vi "Read Configuration File.vi"(8 "error in (no error)":errorcluster, 10 "Configuration filepath":string, 11 "TDCManager":T1) -> (0 "error out":errorcluster, 2 "Success?":bool, 3 "TDCManager":T1)   [LabVIEW 2016, in "HPTDC Driver Library.lvlib"]
uses:
  HPTDC Driver Library.lvlib
  Typedefs/TDCManager.ctl
  C:/Users/CRT Controller/CRTC Labview Application/Source/HPTDC Driver Library Folder/Library files/hptdc_net4_3.7.0_x64.dll
  hptdc_net4_3.7.0_x64.dll
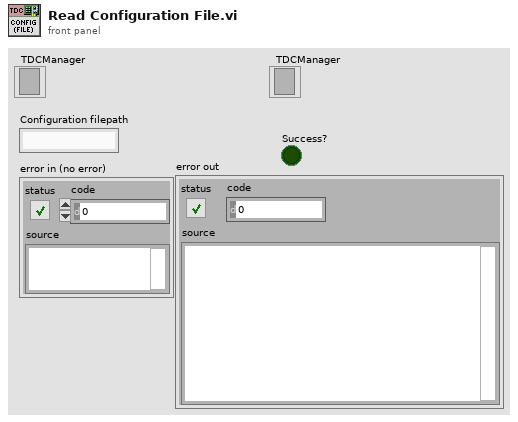
[diagram p1: front panel]
types:
  T1 = typedef "HPTDC Driver Library.lvlib/TDCManager.ctl" = refnum<k24>
  T2 = typedef "Semaphore RefNum" = refnum<k1>
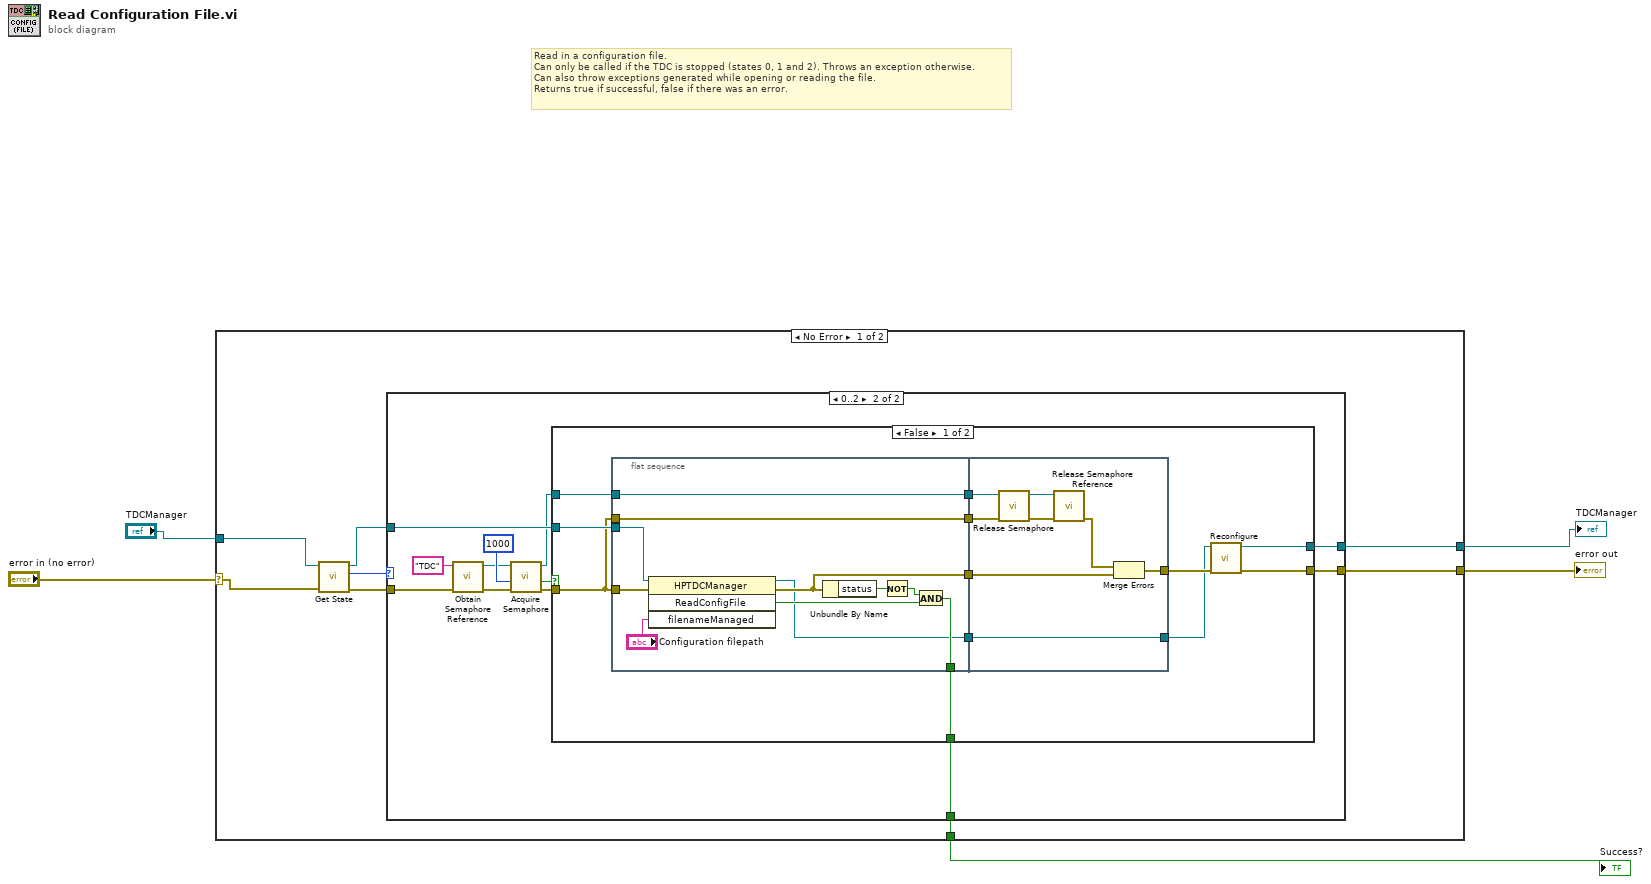
[diagram p0: block diagram]
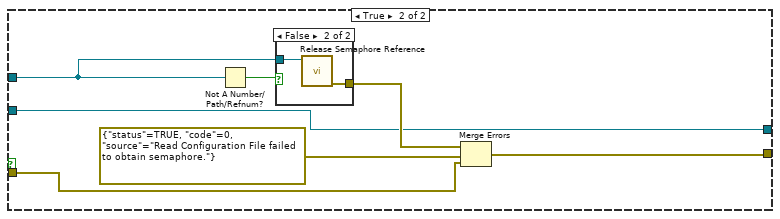
[diagram p3: hidden frame]
diagram:
  # "Read in a configuration file.\nCan only be called if the TDC is stopped (states 0, 1 and 2). Throws an exception otherwise.\nCan also throw exceptions generated while opening or reading the file.\nReturns true if successful, false if there was an error."
  n1 = case shown="No Error" "error in (no error)" {
    selector: "error in (no error)" -> [w6 w68]
    tunnel: [w10 w68] -> w5
    tunnel: [w9 _] -> w4
    tunnel: [w8 w69] -> w3
    tunnel: "TDCManager" -> [w7 w69]
    frame No Error {
      n2 = call "Get State.vi"("error in"=w6, "TDCManager"=w7) -> ("error out"=w11:errorcluster, "State"=w13:i32, "TDCManager"=w12:T1)  [unwired: 6 in, 1 out]
      n3 = case shown="0..2" w13 {
        tunnel: w11 -> [w15 w22]
        tunnel: w12 -> [w14 w27]
        tunnel: [_ w18] -> w9
        tunnel: [w15 w17] -> w10
        tunnel: [w14 w16] -> w8
        frame Default {
        }
        frame 0..2 {
          n4 = call <vilib>:"Obtain Semaphore Reference.vi"("error in (no error)"=w22, "name (unnamed)"="TDC") -> ("error out"=w24:errorcluster, "semaphore"=w25:T2)  [unwired: 3 in, 1 out]
          n5 = call <vilib>:"Acquire Semaphore.vi"("error in (no error)"=w24, "ms timeout (-1)"=1000, "semaphore"=w25) -> ("error out"=w20:errorcluster, "timed out"=w21:bool, "semaphore out"=w19:T2)  [unwired: 2 in]
          n6 = case shown="False" w21 {
            tunnel: w27 -> [w39 w59]
            tunnel: w20 -> [w36 w60]
            tunnel: w19 -> [w34 w61]
            tunnel: [w33 _] -> w18
            tunnel: [w31 w62] -> w17
            tunnel: [w30 w59] -> w16
            frame False {
              n7 = flat-sequence {
                tunnel: w36 -> [w50]
                tunnel: w39 -> [w49]
                tunnel: [w48] -> w38
                tunnel: w36 -> [w43]
                tunnel: [w43] -> w37
                tunnel: [w42] -> w35
                tunnel: w34 -> [w42]
                tunnel: [w41] -> w33
                tunnel: [w40] -> w29
                tunnel: w38 -> [w58]
                tunnel: w37 -> [w55]
                tunnel: w35 -> [w53]
                tunnel: [w52] -> w32
                tunnel: w29 -> [w51]
                tunnel: [w51] -> w28
                frame #0 {
                  n8 = invoke class="HPTDCManager" method="ReadConfigFile"(reference=w49, error in=w50, "filenameManaged"="Configuration filepath") -> (reference out=w40:T1, error out=w48:errorcluster, "ReadConfigFile"=w47:bool)  [unwired: 1 in, 1 out]
                  n9 = Unbundle By Name(w48) -> ("status"=w46:bool)
                  n10 = Not(x=w46) -> (.not. x?=w45:bool)
                  n11 = And(x=w45, y=w47) -> (x .and. y?=w41:bool)
                }
                frame #1 {
                  n12 = call <vilib>:"Release Semaphore.vi"("error in (no error)"=w55, "semaphore"=w53) -> ("error out"=w56:errorcluster, "semaphore out"=w57:T2)  [unwired: 4 in]
                  n13 = call <vilib>:"Release Semaphore Reference.vi"("error in (no error)"=w56, "semaphore"=w57) -> ("error out"=w54:errorcluster)  [unwired: 8 in, 1 out]
                  n14 = Merge Errors(w54, w58) -> (w52:errorcluster)
                }
              }
              n15 = call "Reconfigure.vi"("error in (no error)"=w32, "TDCManager"=w28) -> ("error out"=w31:errorcluster, "TDCManager"=w30:T1)  [unwired: 8 in]
            }
            frame True {
              n16 = Not A Number/Path/Refnum?(number/path/refnum=w61) -> (NaN/Path/Refnum?=w65:bool)
              n17 = case shown="False" w65 {
                tunnel: [_ w67] -> w64
                tunnel: w61 -> [_ w66]
                frame True {
                }
                frame False {
                  n18 = call <vilib>:"Release Semaphore Reference.vi"("semaphore"=w66) -> ("error out"=w67:errorcluster)  [unwired: 9 in, 1 out]
                }
              }
              n19 = Merge Errors(w64, errorcluster {"status"=TRUE, "code"=0, "source"="Read Configuration File failed to obtain semaphore."} ("error out"), w60) -> (w62:errorcluster)
            }
          }
        }
      }
    }
    frame Error {
    }
  }
  "error out" <- w5
  "Success?" <- w4
  "TDCManager" <- w3
